vi "Latihan 20 (Multiloop Comnection).vi"() -> ()   [LabVIEW 2021]
uses:
  <vilib>/addons/Control Design/_Model Construction/Model Creation.llb/Model Creation SubVI/cd_Create Transfer Function Model.vi
  <vilib>/addons/Control Design/_Model Interconnection/Model Interconnection.llb/Model Interconnection SubVI/cd_Series (TF and TF).vi
  <vilib>/addons/Control Design/_Model Interconnection/Model Interconnection.llb/Model Interconnection SubVI/cd_Feedback (TF and TF).vi
  <vilib>/addons/Control Design/_Utility/Model Viewer.llb/Model Viewer SubVI/cd_Draw Transfer Function Equation (TF).vi
  <vilib>/addons/Control Design/_Model Interconnection/Model Interconnection.llb/Model Interconnection SubVI/cd_Matrix Divide Models (TF and TF).vi
  <vilib>/addons/Control Design/_Model Construction/NI_LinSys_Model Creation.lvlib
  <vilib>/addons/Control Design/_Model Interconnection/NI_CD_Model Interconnection.lvlib
  <vilib>/addons/Control Design/_Utility/NI_CD_Model Viewer.lvlib
panel:
  out "Pole-Zero-gain Model of the System":picture
  out "Transfer Function Model of the System":picture
  in  "Denominator of H2(s)":dbl[](array[numeric])
  in  "Numerator of H2(s)":dbl[](array[numeric])
  in  "Denominator of H3(s)":dbl[](array[numeric])
  in  "Numerator of H3(s)":dbl[](array[numeric])
  in  "Denominator of H1(s)":dbl[](array[numeric])
  in  "Numerator of H1":dbl[](array[numeric])
  in  "Denominator of G4(s)":dbl[](array[numeric])
  in  "Denominator of G3(s)":dbl[](array[numeric])
  in  "Denominator of G2(s)":dbl[](array[numeric])
  in  "Denominator of G1(s)":dbl[](array[numeric])
  in  "Numerator of G4(s)":dbl[](array[numeric])
  in  "Numerator of G3(s)":dbl[](array[numeric])
  in  "Numerator of G2(s)":dbl[](array[numeric])
  in  "Numerator of G1(s)":dbl[](array[numeric])
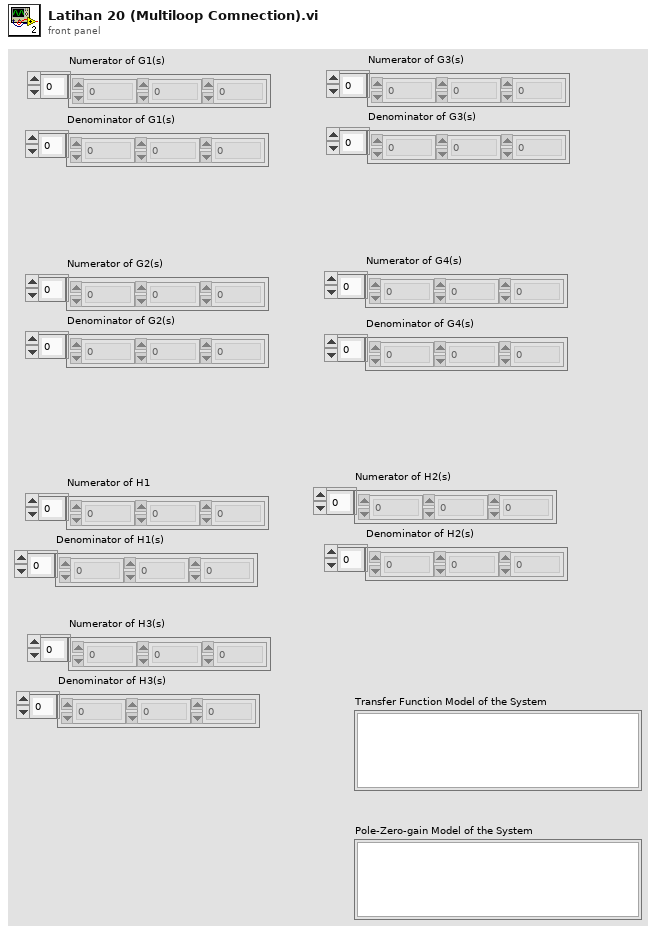
[diagram p1: front panel]
types:
  T1 = typedef "NI_LinSys_Model Typedefs.lvlib/CD Transfer Function Model (MIMO).ctl" = cluster{"properties":T2, "transfer function(s)":T3[][]}
  T2 = typedef "NI_LinSys_Model Typedefs.lvlib/CD General Elements.ctl" = cluster{"Model name":string, "Input names":string[], "Output names":string[], "Input Delays":dbl[], "Output Delays":dbl[], "Sampling Time":dbl, "Notes":string}
  T3 = typedef "NI_LinSys_Model Typedefs.lvlib/CD Transfer Function Model (SISO).ctl" = cluster{"Numerator":dbl[], "Denominator":dbl[], "delay":dbl}
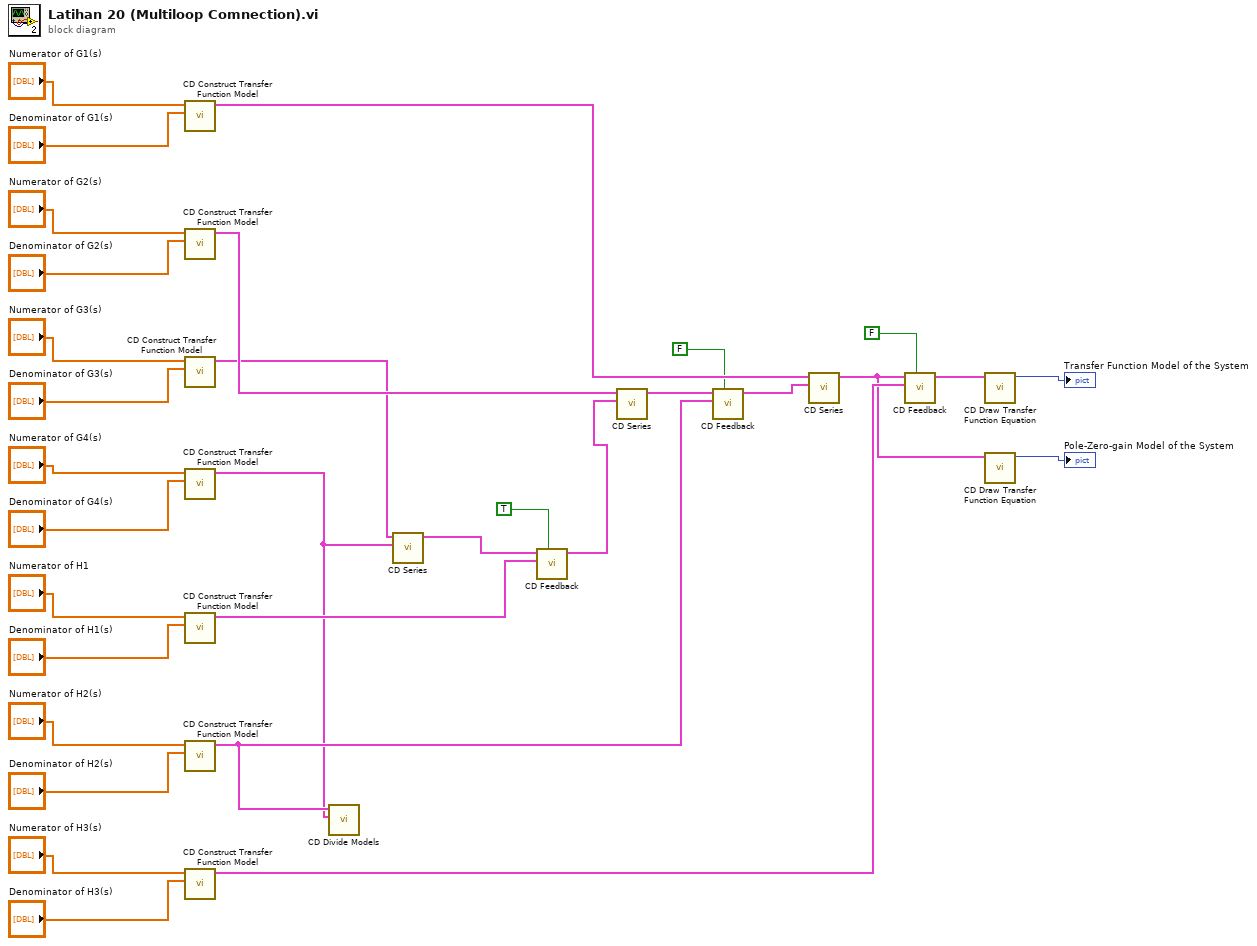
[diagram p0: block diagram]
diagram:
  n1 = call-poly <vilib>:"CD Construct Transfer Function Model.vi"("Denominator"="Denominator of G1(s)", "Numerator"="Numerator of G1(s)") -> ("Transfer Function Model"=w15:T1)  [unwired: 8 in, 1 out]
  n2 = call-poly <vilib>:"CD Construct Transfer Function Model.vi"("Denominator"="Denominator of G2(s)", "Numerator"="Numerator of G2(s)") -> ("Transfer Function Model"=w18:T1)  [unwired: 8 in, 1 out]
  n3 = call-poly <vilib>:"CD Construct Transfer Function Model.vi"("Denominator"="Denominator of G3(s)", "Numerator"="Numerator of G3(s)") -> ("Transfer Function Model"=w12:T1)  [unwired: 8 in, 1 out]
  n4 = call-poly <vilib>:"CD Construct Transfer Function Model.vi"("Denominator"="Denominator of G4(s)", "Numerator"="Numerator of G4(s)") -> ("Transfer Function Model"=w2:T1)  [unwired: 8 in, 1 out]
  n5 = call-poly <vilib>:"CD Construct Transfer Function Model.vi"("Denominator"="Denominator of H1(s)", "Numerator"="Numerator of H1") -> ("Transfer Function Model"=w11:T1)  [unwired: 8 in, 1 out]
  n6 = call-poly <vilib>:"CD Construct Transfer Function Model.vi"("Denominator"="Denominator of H2(s)", "Numerator"="Numerator of H2(s)") -> ("Transfer Function Model"=w3:T1)  [unwired: 8 in, 1 out]
  n7 = call-poly <vilib>:"CD Construct Transfer Function Model.vi"("Denominator"="Denominator of H3(s)", "Numerator"="Numerator of H3(s)") -> ("Transfer Function Model"=w9:T1)  [unwired: 8 in, 1 out]
  n8 = call-poly <vilib>:"CD Divide Models.vi"("Model 2"=w2, "Model 1"=w3) -> ()  [unwired: 8 in, 2 out]
  n9 = call-poly <vilib>:"CD Series.vi"("Model 2"=w2, "Model 1"=w12) -> ("Series Model"=w13:T1)  [unwired: 8 in, 1 out]
  n10 = call-poly <vilib>:"CD Feedback.vi"("Feedback Sign"=TRUE, "Model 2"=w11, "Model 1"=w13) -> ("Closed-Loop Model"=w14:T1)  [unwired: 7 in, 1 out]
  n11 = call-poly <vilib>:"CD Series.vi"("Model 2"=w14, "Model 1"=w18) -> ("Series Model"=w17:T1)  [unwired: 8 in, 1 out]
  n12 = call-poly <vilib>:"CD Feedback.vi"("Feedback Sign"=FALSE, "Model 2"=w3, "Model 1"=w17) -> ("Closed-Loop Model"=w16:T1)  [unwired: 7 in, 1 out]
  n13 = call-poly <vilib>:"CD Series.vi"("Model 2"=w16, "Model 1"=w15) -> ("Series Model"=w5:T1)  [unwired: 8 in, 1 out]
  n14 = call-poly <vilib>:"CD Feedback.vi"("Feedback Sign"=FALSE, "Model 2"=w9, "Model 1"=w5) -> ("Closed-Loop Model"=w6:T1)  [unwired: 7 in, 1 out]
  n15 = call-poly <vilib>:"CD Draw Transfer Function Equation.vi"("Transfer Function Model"=w6) -> ("Equation"=→"Transfer Function Model of the System":picture)  [unwired: 8 in, 2 out]
  n16 = call-poly <vilib>:"CD Draw Transfer Function Equation.vi"("Transfer Function Model"=w5) -> ("Equation"=→"Pole-Zero-gain Model of the System":picture)  [unwired: 8 in, 2 out]
